vi "UI-电源尾反面标签漏线检测.vi"(8 "error in (no error)":errorcluster caption="错误输入（无错误）", 11 "名称或相对路径":string="Template Program") -> (0 "error in (no error) 2":errorcluster caption="错误输入（无错误）")   [LabVIEW 2017]
uses:
  Picture/SaveButtom.ctl
  Global System.vi
  <vilib>/Utility/xml.llb/Write to XML File(string).vi
panel:
  in  "获取图像":bool
  in  "ROI获取":bool
  in  "创建模板":bool
  in  "保存图像":bool
  out "添加的路径":path
  in  "刷新":bool
  in  "测试按钮":bool
  in  "保存按钮":bool
  in  "Main":enum32{"主参数", "颜色模板匹配参数 ", "测试效果"}(tab)
  in  "UI电源尾反面漏线基础参数":T1={"IsNorImage"=TRUE, "Exposure Values"=100289, "ImagePath"=path "C:/Users/hedongpo/Desktop/514-hdp/Alignment Assemble System/Test Picture/B/3.bmp"} caption="参数界面" {"Exposure Values" scale=0.0..200000.0}
  in  "UI电源尾反面漏线参数":T3={"Rectangle"={"Left"=0, "Top"=0, "Right"=0, "Bottom"=0, "Rotation"=0.0}, "模板路径"=path "C:/Users/delluser001/Desktop/PowerLine Inspect System/Source Code/Template Program/potteryTemplete/Color.png", "Match Mode "=0, "Minimum Match Score "=800.0, "Number of Matches Requested"=1, "Rotation Angle Ranges (degrees)"=[{"Min"=-180.0, "Max"=180.0}], "Color Sensitivity "=0, "Match Offset"={"X"=0.0, "Y"=0.0}, "Color Score Weight "=500.0, "Search Strategy "=0, "Subpixel Accuracy "=FALSE, "Range (Threshold 1)"={"Lower value"=148.0, "Upper value"=255.0}} {"Rectangle"."Rotation" format="%.2f"; "Rectangle"."Left" scale=0.0..1024.0; "Rectangle"."Right" scale=0.0..1024.0; "Search Strategy" items=["Conservative", "Balance", "Aggressive", "Very Aggressive"]; "Color Sensitivity" items=["Low Sensitivity", "Medium Sensitivity", "High Sensitivity"]; "Match Mode" items=["Shift Invariant", "Rotation Invariant"]}
  out "原始图像":T4(plugin-control)
  out "x = 0?":bool
  out "路径输出":path
  in  "Vision Paramter Save Buttom":T5
  out "system time":string
  in  "取消按钮":bool
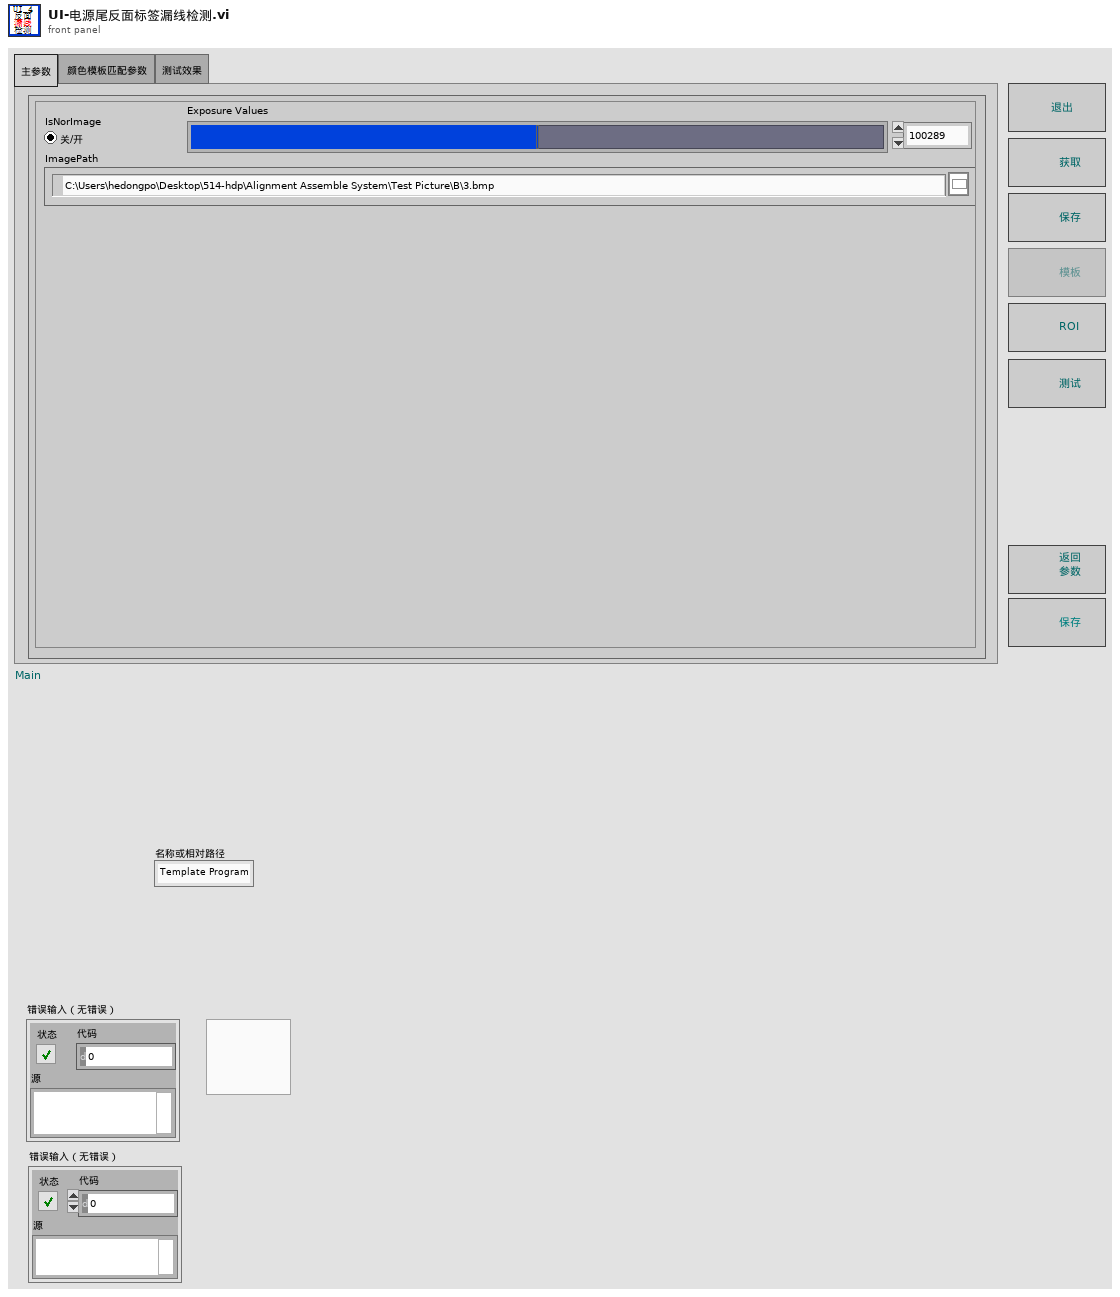
[diagram p1: front panel]
types:
  T1 = cluster{"IsNorImage":bool, "Exposure Values":u32, "ImagePath":path}
  T2 = typedef "IMAQ Rectangle" = cluster{"Left":i32, "Top":i32, "Right":i32, "Bottom":i32, "Rotation":dbl}
  T3 = cluster{"Rectangle":T2, "模板路径":path, "Match Mode ":u32, "Minimum Match Score ":sgl, "Number of Matches Requested":i32, "Rotation Angle Ranges (degrees)":cluster{"Min":sgl, "Max":sgl}[], "Color Sensitivity ":u32, "Match Offset":cluster{"X":sgl, "Y":sgl}, "Color Score Weight ":sgl, "Search Strategy ":u32, "Subpixel Accuracy ":bool, "Range (Threshold 1)":cluster{"Lower value":sgl, "Upper value":sgl}}
  T4 = typedef "IMAQ Image.ctl" = refnum<image>
  T5 = typedef "SaveButtom.ctl" = bool
  T6 = cluster{"index":i32, "this vi":refnum<vi>, "error out":errorcluster}
  T7 = cluster{"master data":string, "priority":u16, "secondary data":string[]}
  T8 = cluster{"case name":string[], "queue array":refnum<queue>[]}
  T9 = cluster{"Global Rectangle":i32[], "Contours":cluster{"Contour Type":u32, "ROI Type":u32, "Points":i32[]}[]}
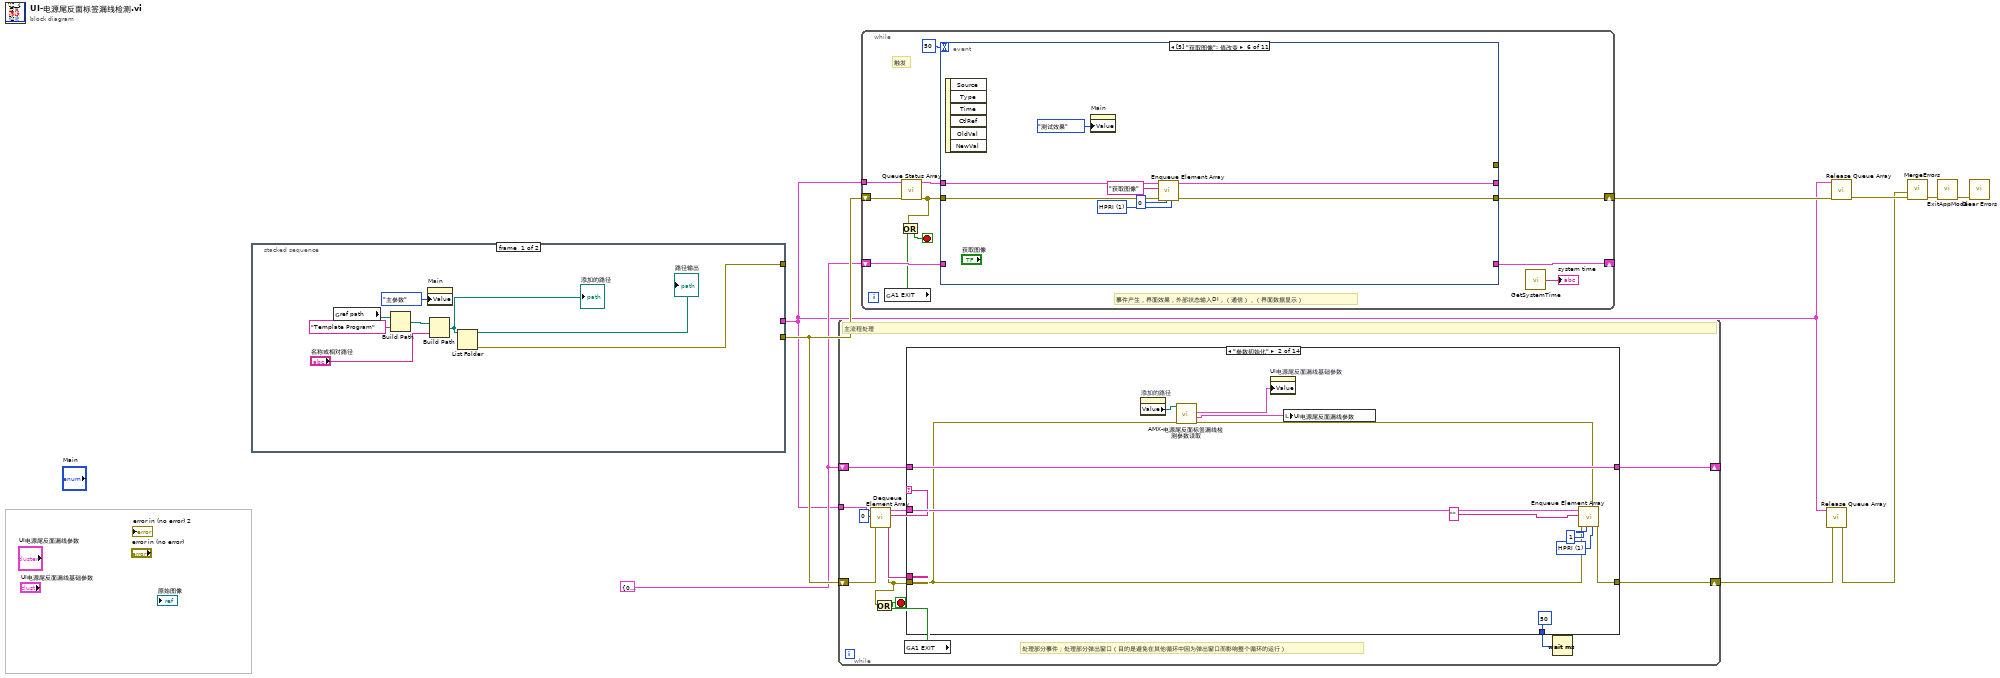
[diagram p0: block diagram]
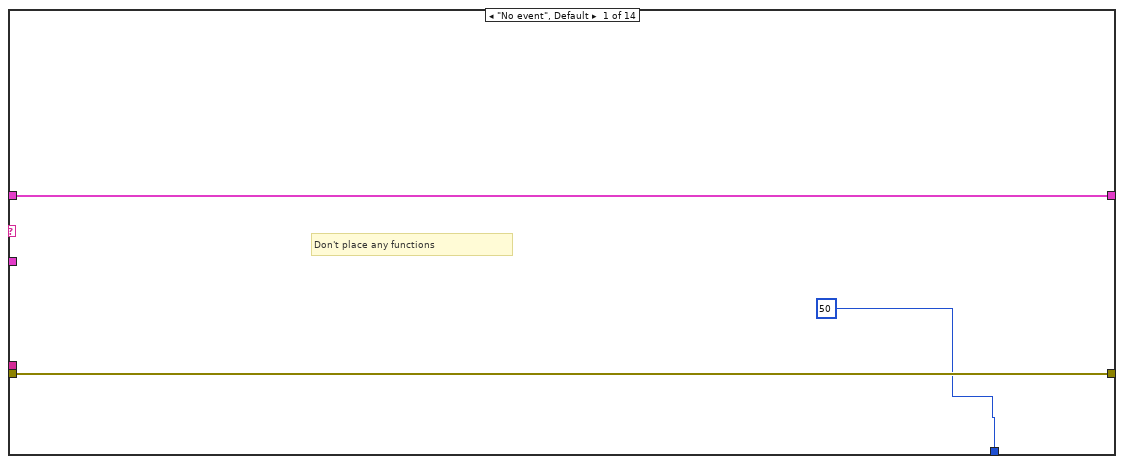
[diagram p2: hidden frame]
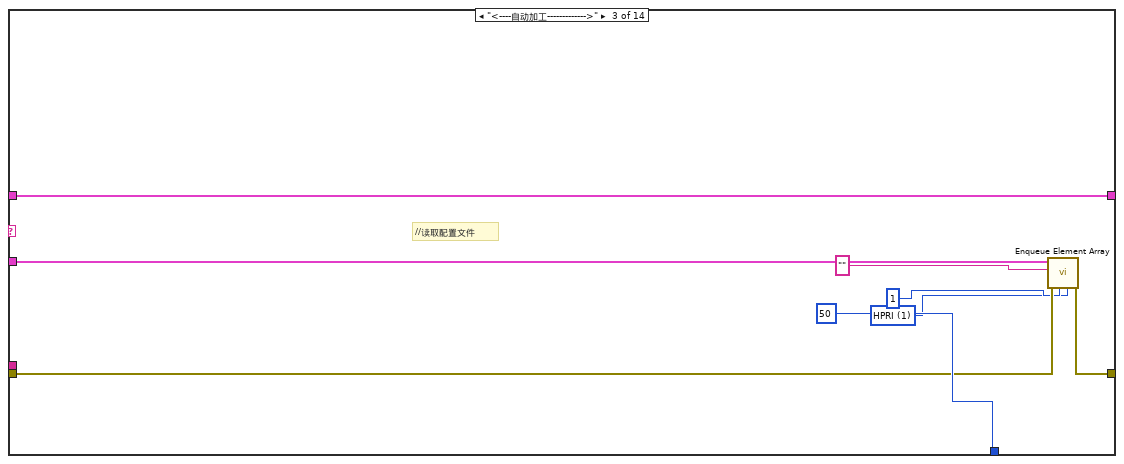
[diagram p3: hidden frame]
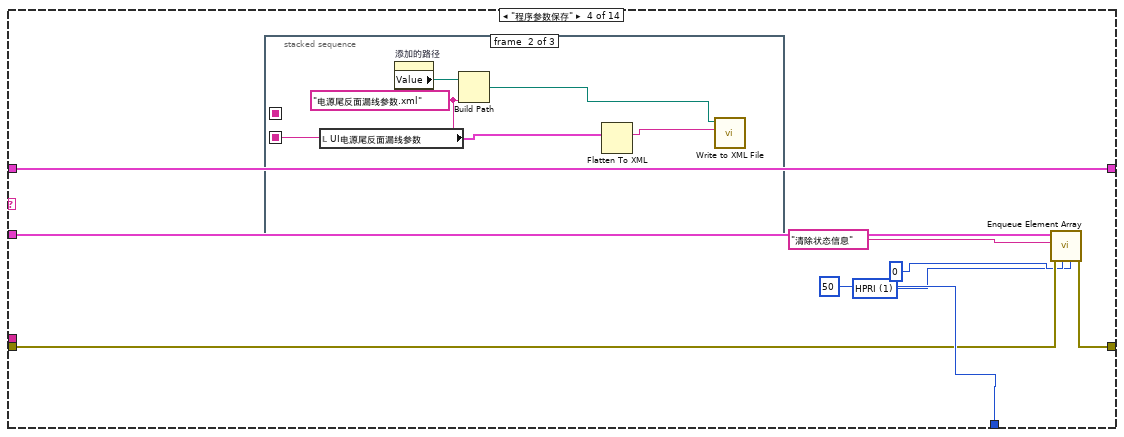
[diagram p4: hidden frame]
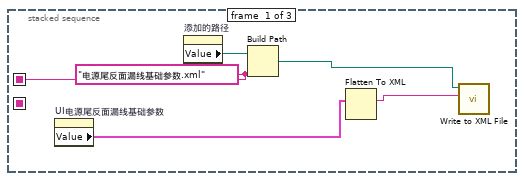
[diagram p5: hidden frame]
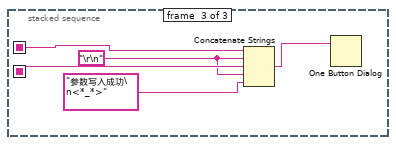
[diagram p6: hidden frame]
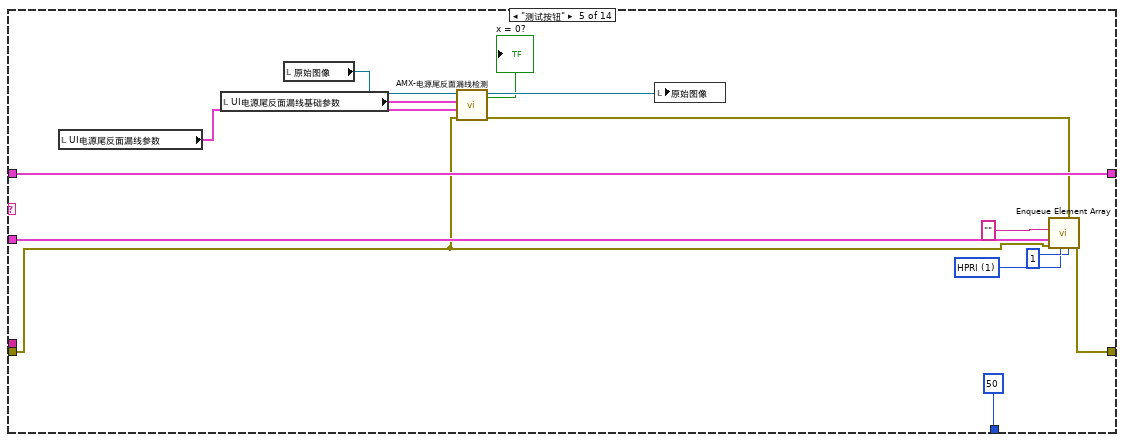
[diagram p7: hidden frame]
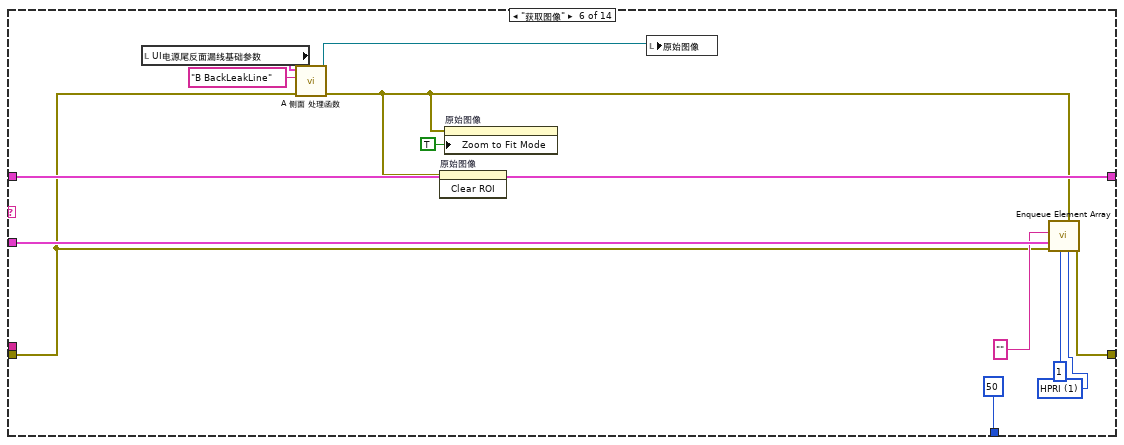
[diagram p8: hidden frame]
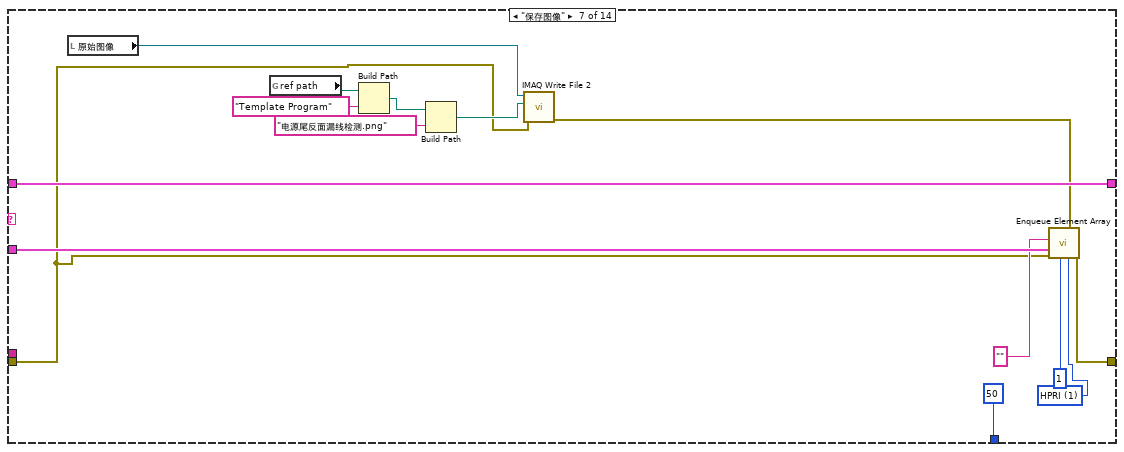
[diagram p9: hidden frame]
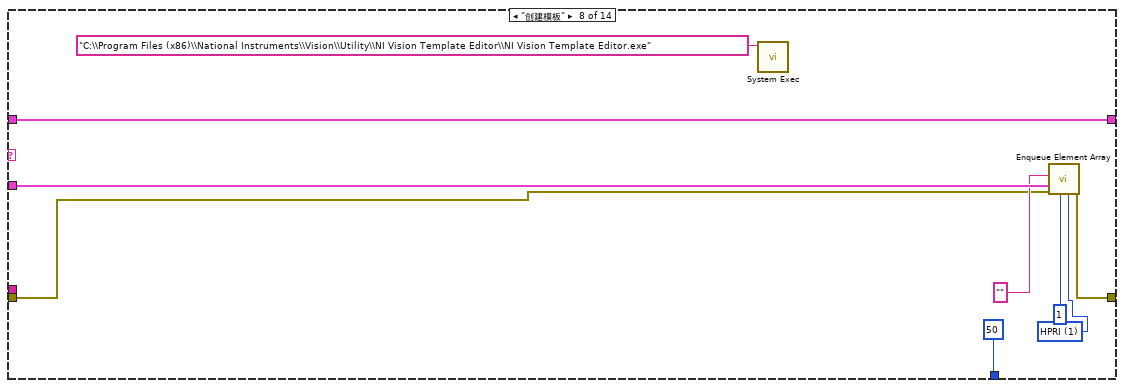
[diagram p10: hidden frame]
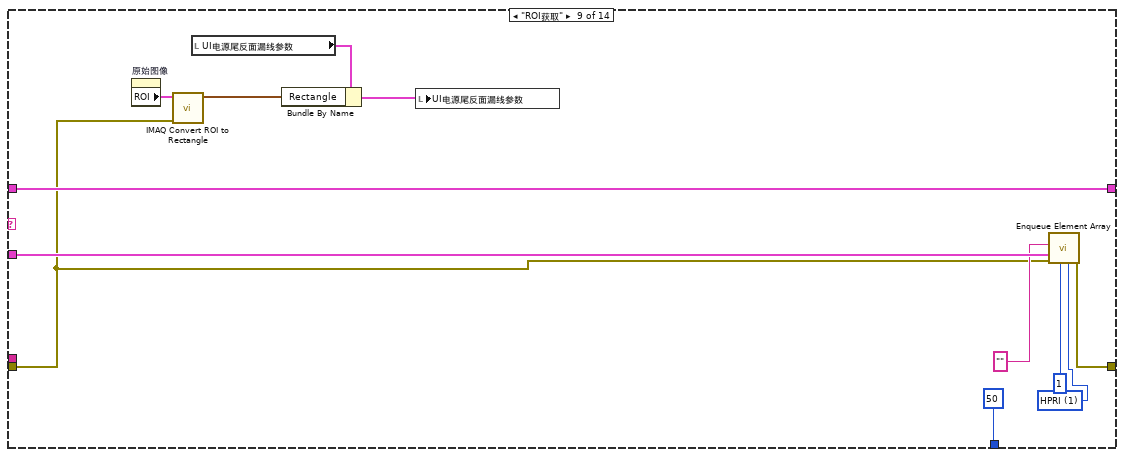
[diagram p11: hidden frame]
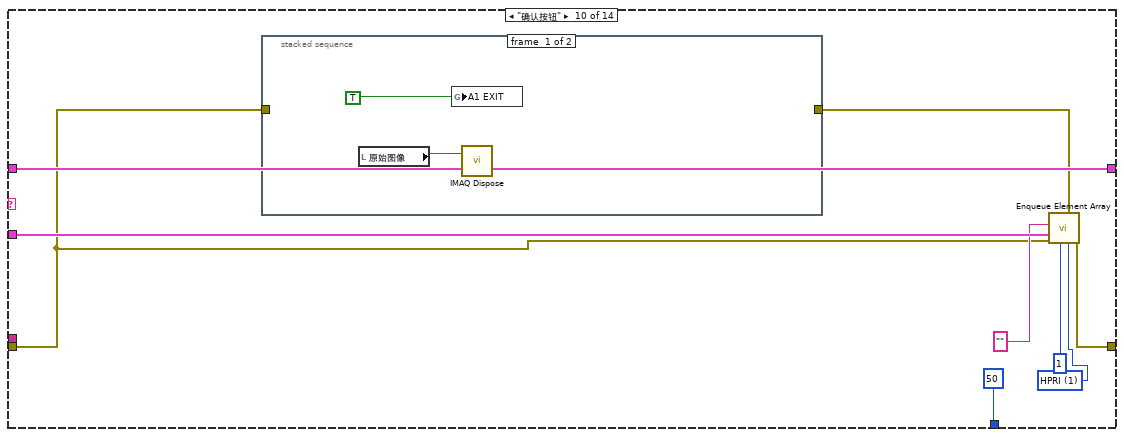
[diagram p12: hidden frame]
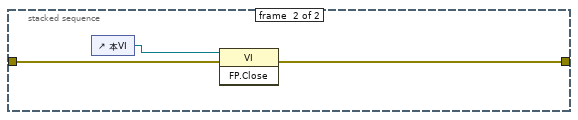
[diagram p13: hidden frame]
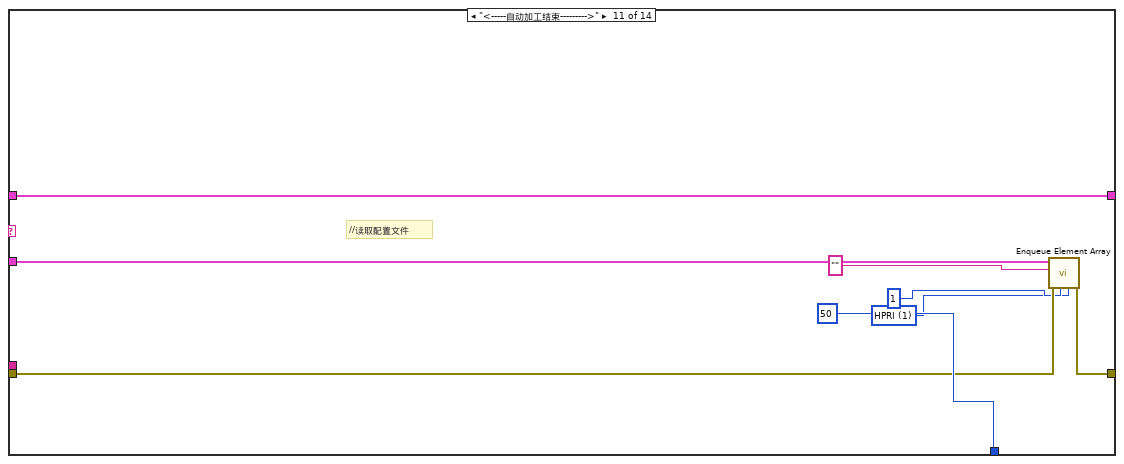
[diagram p14: hidden frame]
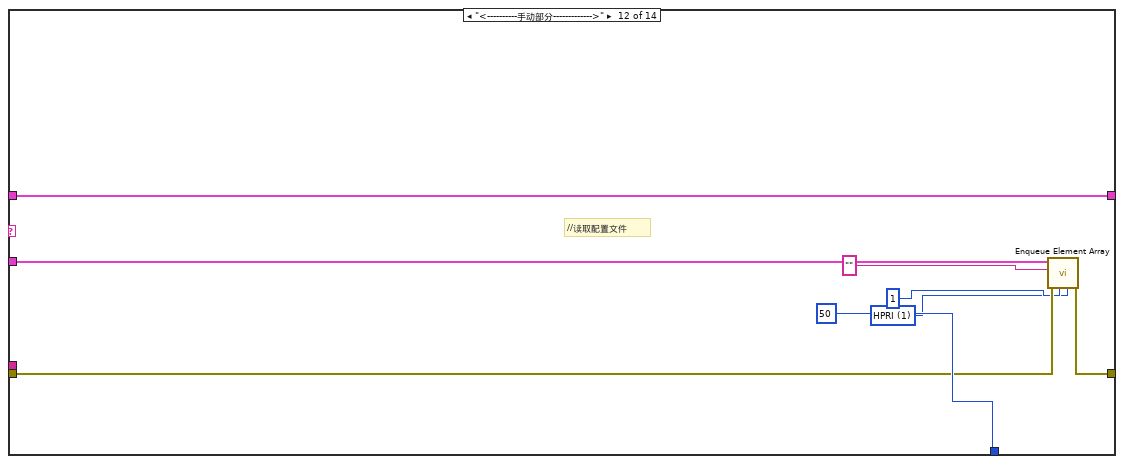
[diagram p15: hidden frame]
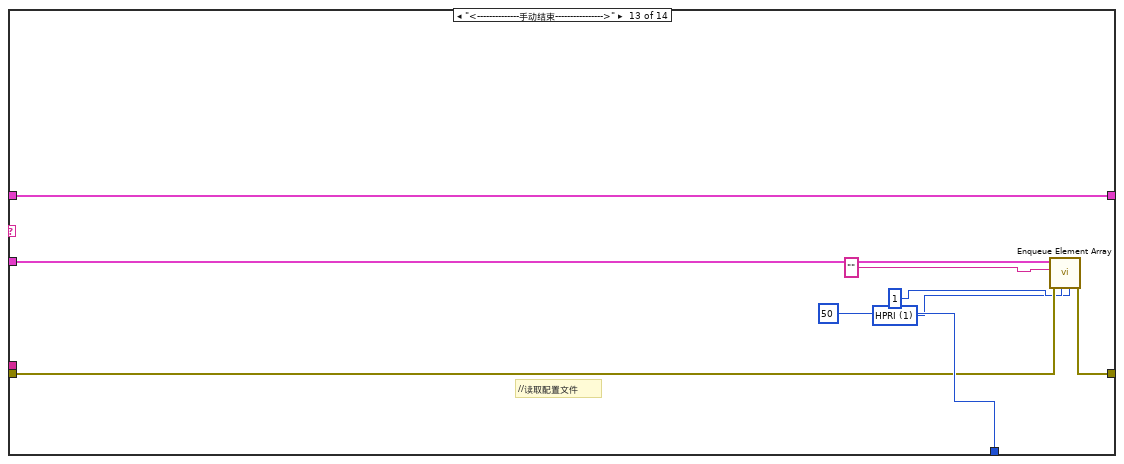
[diagram p16: hidden frame]
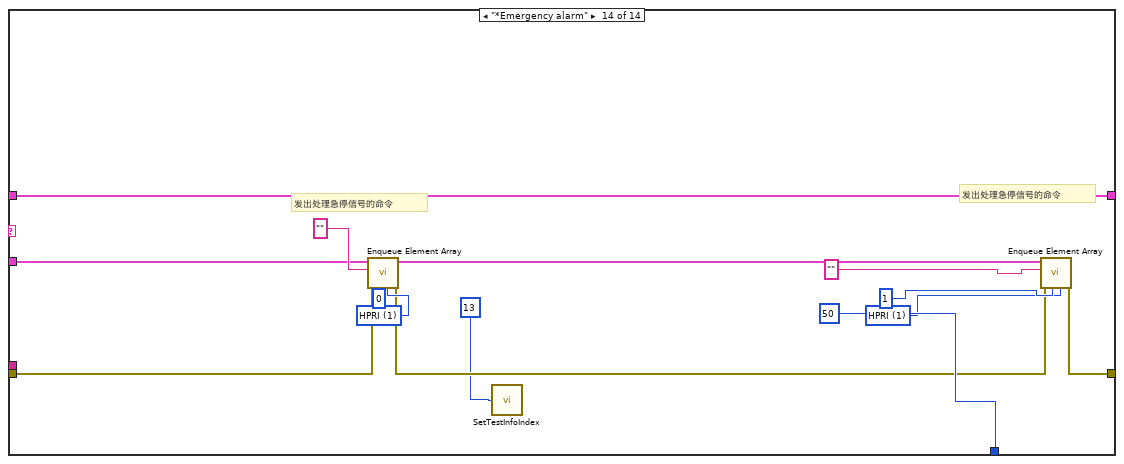
[diagram p17: hidden frame]
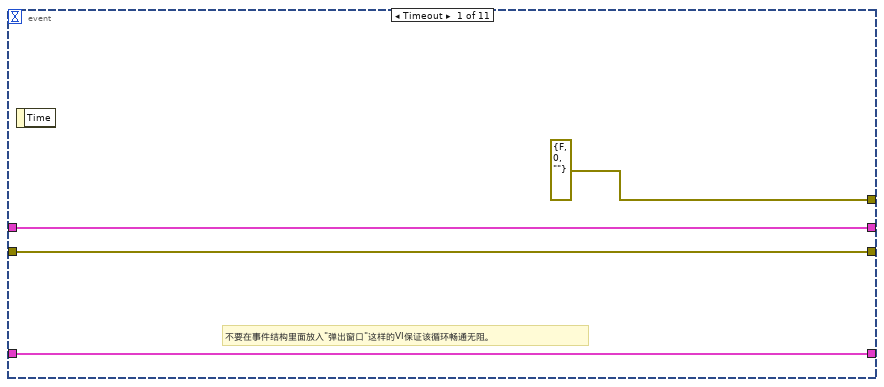
[diagram p18: hidden frame]
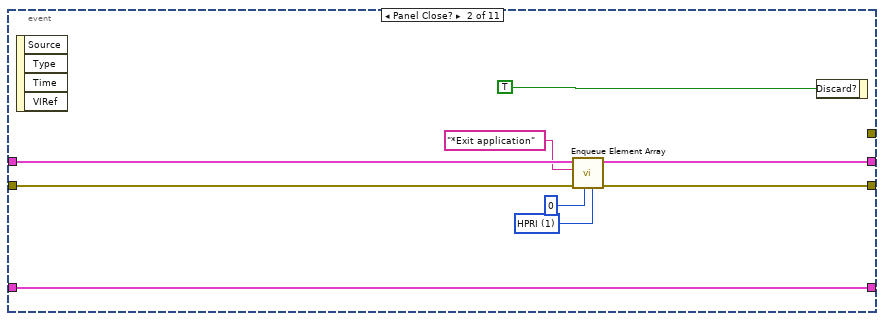
[diagram p19: hidden frame]
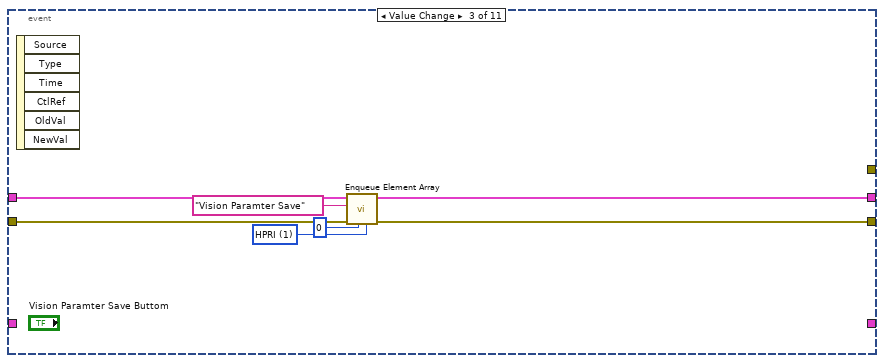
[diagram p20: hidden frame]
diagram:
  w4 = T6 {"index"=0, "this vi"=refnum, "error out"={"status"=FALSE, "code"=0, "source"=""}} ("parameter buffer")
  n1 = stacked-sequence {
    tunnel: [w16 _] -> _
    tunnel: [_ w19] -> w5
    tunnel: [_ w18] -> w1
    frame #0 {
      n2 = global read "Global System.vi" "ref path"() -> (w14:path)
      n3 = Build Path(base path=w14, name or relative path="Template Program" ("名称或相对路径")) -> (appended path=w12:path)
      n4 = property on="Main" class="TabCtl (严格)"("Value"=enum32{"主参数", "颜色模板匹配参数 ", "测试效果"}."主参数" ("Main")) -> ()  [unwired: 2 in, 2 out]
      n5 = Build Path(base path=w12, name or relative path="名称或相对路径") -> (appended path=w10:path)
      "添加的路径" <- w10
      n6 = List Folder(path=w10) -> (path out=→"路径输出":path, error out=w16:errorcluster)  [unwired: 3 in, 2 out]
    }
    frame #1 {
      w27 = string[] ["comm queue1", "data queue 11", "data queue 12", "data queue 13", "data queue 14"]  # queue name
      w28 = 4  # queue num
      w29 = T7 {"master data"="", "priority"=0, "secondary data"=[]}  # element data type
      n7 = call "Obtain Queue Array.vi"("queue name"=w27, "element data type"=w29, "queue num"=w28) -> ("error out"=w23:errorcluster, "queue out"=w24:T8)  [unwired: 2 in, 1 out]
      n8 = call "Enqueue Element Array.vi"("queue index"=0, "error in"=w23, "master data"="参数初始化", "queue in"=w24) -> ("error out"=w22:errorcluster, "queue out"=w21:T8)  [unwired: 6 in]
      n9 = disable-structure shown="启用" {
        disable-tunnel: w22 -> [w35 w36]
        disable-tunnel: w21 -> [w34 w37]
        disable-tunnel: "Loading Variable" ("master data") -> [w33 _]
        disable-tunnel: [w31 w36] -> w19
        disable-tunnel: [w30 w37] -> w18
        frame Disabled {
          n10 = call "Enqueue Element Array.vi"("queue index"=12, "error in"=w35, "master data"=w33, "queue in"=w34) -> ("error out"=w31:errorcluster, "queue out"=w30:T8)  [unwired: 6 in]
        }
        frame Enabled {
        }
      }
    }
  }
  n11 = while {
    shift-right: [w50] -> w3
    shift-left: w5 -> [w41]
    shift-right: [w47] -> _
    shift-left: w4 -> [w48]
    tunnel: w1 -> [w43]
    stop <- w38 stop-if-true
    # "处理部分事件；处理部分弹出窗口（目的是避免在其他循环中因为弹出窗口而影响整个循环的运行）"
    # "主流程处理"
    n12 = call "Dequeue Element Array.vi"("queue in"=w43, "queue index"=0, "error in"=w41) -> ("queue out"=w46:T8, "master data"=w45:string, "secondary data"=w44:string[], "error out"=w40:errorcluster)  [unwired: 2 in, 1 out]
    n13 = global read "Global System.vi" "A1 EXIT"() -> (w39:bool)
    n14 = Or(x=w40, y=w39) -> (x .or. y?=w38:bool)
    n15 = case shown="\"参数初始化\"" w45 {
      tunnel: w46 -> [_ w64 w72 w74 w109 w122 w137 w146 w158 w167 w180 w188 w196 w202]
      tunnel: w40 -> [w52 w57 w68 w78 w102 w113 w124 w140 w151 w161 w176 w184 w192 w199]
      tunnel: [w52 w63 w71 w80 w108 w121 w136 w145 w157 w166 w179 w187 w195 w210] -> w50
      tunnel: [50 50 50 50 50 50 50 50 50 50 50 50 50 50] -> w49
      tunnel: w48 -> [w53 w59 w69 w75 w104 w117 w132 w141 w153 w162 w177 w185 w193 w208]
      tunnel: [w53 w59 w69 w75 w104 w117 w132 w141 w153 w162 w177 w185 w193 w208] -> w47
      tunnel: w44 -> [_ _ _ _ _ _ _ _ _ _ _ _ _ _]
      frame "No event", Default {
        # "Don't place any functions"
      }
      frame "参数初始化" {
        w60 = u16 1 items=["HPRI"=1, "LPRI"=0] ("priority")
        n16 = property on="添加的路径" class="Path"() -> ("Value"=w58:path)  [unwired: 2 in, 2 out]
        n17 = call "AMX-电源尾反面标签漏线检测参数读取.vi"("error in (no error)"=w57, "基路径"=w58) -> ("error out"=w55:errorcluster, "UI电源尾反面漏线参数"=w54:T3, "UI电源尾反面漏线基础参数"=w56:T1)  [unwired: 6 in]
        n18 = property on="UI电源尾反面漏线基础参数" class="Clust (严格)"("Value"=w56) -> ()  [unwired: 2 in, 2 out]
        n19 = local write "UI电源尾反面漏线参数"(w54) -> ()
        n20 = call "Enqueue Element Array.vi"("priority"=w60, "device error in"=w55, "queue index"=1, "error in"=w57, "master data"="" ("Element 1"), "queue in"=w64) -> ("error out"=w63:errorcluster)  [unwired: 4 in, 1 out]
      }
      frame "<----自动加工------------->" {
        w66 = u16 1 items=["HPRI"=1, "LPRI"=0] ("priority")
        # "//读取配置文件"
        n21 = call "Enqueue Element Array.vi"("priority"=w66, "queue index"=1, "error in"=w68, "master data"="" ("Element 1"), "queue in"=w72) -> ("error out"=w71:errorcluster)  [unwired: 5 in, 1 out]
      }
      frame "程序参数保存" {
        w76 = u16 1 items=["HPRI"=1, "LPRI"=0] ("priority")
        n22 = stacked-sequence {
          seq-local: [w82 _ _] -> [_ _ w95]
          seq-local: [_ w88 _] -> [_ _ w93]
          frame #0 {
            w82 = "电源尾反面漏线基础参数.xml" ("名称或相对路径")
            n23 = property on="UI电源尾反面漏线基础参数" class="Clust (严格)"() -> ("Value"=w85:T1)  [unwired: 2 in, 2 out]
            n24 = property on="添加的路径" class="Path"() -> ("Value"=w86:path)  [unwired: 2 in, 2 out]
            n25 = Build Path(base path=w86, name or relative path=w82) -> (appended path=w83:path)
            n26 = Flatten To XML(anything=w85) -> (xml string=w84:string)
            n27 = call-poly <vilib>:"Write to XML File.vi"("XML Input"=w84, "XML File Path"=w83) -> ()  [unwired: 7 in, 3 out]
          }
          frame #1 {
            w88 = "电源尾反面漏线参数.xml" ("名称或相对路径")
            n28 = local read "UI电源尾反面漏线参数"() -> (w87:T3)
            n29 = property on="添加的路径" class="Path"() -> ("Value"=w91:path)  [unwired: 2 in, 2 out]
            n30 = Build Path(base path=w91, name or relative path=w88) -> (appended path=w89:path)
            n31 = Flatten To XML(anything=w87) -> (xml string=w90:string)
            n32 = call-poly <vilib>:"Write to XML File.vi"("XML Input"=w90, "XML File Path"=w89) -> ()  [unwired: 7 in, 3 out]
          }
          frame #2 {
            w92 = "\r\n"
            n33 = Concatenate Strings(w95, w92, w93, w92, "参数写入成功\n<*_*>" ("消息")) -> (w94:string)
            n34 = One Button Dialog(message=w94) -> ()  [unwired: 1 in, 1 out]
          }
        }
        n35 = call "Enqueue Element Array.vi"("priority"=w76, "queue index"=0, "error in"=w78, "master data"="清除状态信息" ("Element 1"), "queue in"=w74) -> ("error out"=w80:errorcluster)  [unwired: 5 in, 1 out]
      }
      frame "测试按钮" {
        w105 = u16 1 items=["HPRI"=1, "LPRI"=0] ("priority")
        n36 = local read "UI电源尾反面漏线参数"() -> (w98:T3)
        n37 = local read "UI电源尾反面漏线基础参数"() -> (w103:T1)
        n38 = local read "原始图像"() -> (w100:T4)
        n39 = call "AMX-电源尾反面漏线检测.vi"("error in (no error)"=w102, "UI电源线正面漏线参数"=w98, "电源线正面标签1基础参数"=w103, "Image in"=w100) -> ("error out"=w99:errorcluster, "Image out"=w101:T4, "x = 0?"=→"x = 0?":bool)  [unwired: 5 in]
        n40 = local write "原始图像"(w101) -> ()
        n41 = call "Enqueue Element Array.vi"("priority"=w105, "device error in"=w99, "queue index"=1, "error in"=w102, "master data"="" ("Element 1"), "queue in"=w109) -> ("error out"=w108:errorcluster)  [unwired: 4 in, 1 out]
      }
      frame "获取图像" {
        w118 = u16 1 items=["HPRI"=1, "LPRI"=0] ("priority")
        n42 = local read "UI电源尾反面漏线基础参数"() -> (w115:T1)
        n43 = call "A 侧面 处理函数.vi"("error in (no error)"=w113, "Image Name"="B BackLeakLine", "ParamsUI"=w115) -> ("error out"=w111:errorcluster, "Image out"=w114:T4)  [unwired: 5 in, 2 out]
        n44 = invoke on="原始图像" class="ImageControl" method="Clear ROI"(error in=w111) -> ()  [unwired: 2 in, 3 out]
        n45 = property on="原始图像" class="ImageControl"(error in=w111, "Zoom to Fit Mode"=TRUE) -> ()  [unwired: 1 in, 2 out]
        n46 = local write "原始图像"(w114) -> ()
        n47 = call "Enqueue Element Array.vi"("priority"=w118, "device error in"=w111, "queue index"=1, "error in"=w113, "master data"="" ("Element 1"), "queue in"=w122) -> ("error out"=w121:errorcluster)  [unwired: 4 in, 1 out]
      }
      frame "保存图像" {
        w133 = u16 1 items=["HPRI"=1, "LPRI"=0] ("priority")
        n48 = local read "原始图像"() -> (w125:T4)
        n49 = global read "Global System.vi" "ref path"() -> (w131:path)
        n50 = Build Path(base path=w131, name or relative path="Template Program" ("名称或相对路径")) -> (appended path=w129:path)
        n51 = Build Path(base path=w129, name or relative path="电源尾反面漏线检测.png" ("名称或相对路径")) -> (appended path=w127:path)
        n52 = call-poly "IMAQ Write File 2"("error in (no error)"=w124, "File Path"=w127, "Image"=w125) -> ("error out"=w126:errorcluster)  [unwired: 7 in, 1 out]
        n53 = call "Enqueue Element Array.vi"("priority"=w133, "device error in"=w126, "queue index"=1, "error in"=w124, "master data"="" ("Element 1"), "queue in"=w137) -> ("error out"=w136:errorcluster)  [unwired: 4 in, 1 out]
      }
      frame "创建模板" {
        w142 = u16 1 items=["HPRI"=1, "LPRI"=0] ("priority")
        n54 = call <vilib>:"System Exec.vi"("command line"="C:\\Program Files (x86)\\National Instruments\\Vision\\Utility\\NI Vision Template Editor\\NI Vision Template Editor.exe") -> ()  [unwired: 7 in, 4 out]
        n55 = call "Enqueue Element Array.vi"("priority"=w142, "queue index"=1, "error in"=w140, "master data"="" ("Element 1"), "queue in"=w146) -> ("error out"=w145:errorcluster)  [unwired: 5 in, 1 out]
      }
      frame "ROI获取" {
        w154 = u16 1 items=["HPRI"=1, "LPRI"=0] ("priority")
        n56 = property on="原始图像" class="ImageControl"() -> ("ROI"=w152:T9)  [unwired: 2 in, 2 out]
        n57 = call "IMAQ Convert ROI to Rectangle"("error in (no error)"=w151, "ROI Descriptor"=w152) -> ("Rectangle"=w149:T2)  [unwired: 7 in, 1 out]
        n58 = local read "UI电源尾反面漏线参数"() -> (w150:T3)
        n59 = Bundle By Name(cluster=w150, "Rectangle"=w149) -> (w148:T3)
        n60 = local write "UI电源尾反面漏线参数"(w148) -> ()
        n61 = call "Enqueue Element Array.vi"("priority"=w154, "queue index"=1, "error in"=w151, "master data"="" ("Element 1"), "queue in"=w158) -> ("error out"=w157:errorcluster)  [unwired: 5 in, 1 out]
      }
      frame "确认按钮" {
        w163 = u16 1 items=["HPRI"=1, "LPRI"=0] ("priority")
        n62 = stacked-sequence {
          tunnel: w161 -> [_ w172]
          tunnel: [_ w171] -> w160
          frame #0 {
            n63 = local read "原始图像"() -> (w169:T4)
            n64 = global write "Global System.vi" "A1 EXIT"(TRUE ("EXIT")) -> ()
            n65 = call "IMAQ Dispose"("Image"=w169) -> ()  [unwired: 5 in, 1 out]
          }
          frame #1 {
            n66 = control-ref of="本VI"() -> (w173:refnum<vi>)
            n67 = invoke class="VI" method="FP.Close"(reference=w173, error in=w172) -> (error out=w171:errorcluster)  [unwired: 1 in, 2 out]
          }
        }
        n68 = call "Enqueue Element Array.vi"("priority"=w163, "device error in"=w160, "queue index"=1, "error in"=w161, "master data"="" ("Element 1"), "queue in"=w167) -> ("error out"=w166:errorcluster)  [unwired: 4 in, 1 out]
      }
      frame "<-----自动加工结束--------->" {
        w174 = u16 1 items=["HPRI"=1, "LPRI"=0] ("priority")
        # "//读取配置文件"
        n69 = call "Enqueue Element Array.vi"("priority"=w174, "queue index"=1, "error in"=w176, "master data"="" ("Element 1"), "queue in"=w180) -> ("error out"=w179:errorcluster)  [unwired: 5 in, 1 out]
      }
      frame "<----------手动部分------------->" {
        w182 = u16 1 items=["HPRI"=1, "LPRI"=0] ("priority")
        # "//读取配置文件"
        n70 = call "Enqueue Element Array.vi"("priority"=w182, "queue index"=1, "error in"=w184, "master data"="" ("Element 1"), "queue in"=w188) -> ("error out"=w187:errorcluster)  [unwired: 5 in, 1 out]
      }
      frame "<--------------手动结束---------------->" {
        w190 = u16 1 items=["HPRI"=1, "LPRI"=0] ("priority")
        # "//读取配置文件"
        n71 = call "Enqueue Element Array.vi"("priority"=w190, "queue index"=1, "error in"=w192, "master data"="" ("Element 1"), "queue in"=w196) -> ("error out"=w195:errorcluster)  [unwired: 5 in, 1 out]
      }
      frame "*Emergency alarm" {
        w205 = u16 1 items=["HPRI"=1, "LPRI"=0] ("priority")
        w206 = u16 1 items=["HPRI"=1, "LPRI"=0] ("priority")
        # "发出处理急停信号的命令"
        # "发出处理急停信号的命令"
        n72 = call "Enqueue Element Array.vi"("priority"=w205, "queue index"=0, "error in"=w199, "master data"="" ("Element 1"), "queue in"=w202) -> ("error out"=w200:errorcluster, "queue out"=w201:T8)  [unwired: 5 in]
        n73 = call "SetTestInfoIndex.vi"("test info index"=13) -> ()
        n74 = call "Enqueue Element Array.vi"("priority"=w206, "queue index"=1, "error in"=w200, "master data"="" ("Element 1"), "queue in"=w201) -> ("error out"=w210:errorcluster)  [unwired: 5 in, 1 out]
      }
    }
    n75 = Wait (ms)(milliseconds to wait=w49) -> ()  [unwired: 1 out]
  }
  n76 = while {
    shift-right: [w215] -> w6
    shift-left: w5 -> [w219]
    shift-right: [w217] -> _
    shift-left: w4 -> [w218]
    tunnel: w1 -> [w221]
    stop <- w212 stop-if-true
    # "触发"
    # "事件产生，界面效果，外部状态输入DI，（通信），（界面数据显示）"
    n77 = global read "Global System.vi" "A1 EXIT"() -> (w213:bool)
    n78 = call "Queue Status Array.vi"("error in (no error)"=w219, "queue in"=w221) -> ("error out"=w214:errorcluster, "queue out"=w216:T8)  [unwired: 4 in]
    n79 = Or(x=w214, y=w213) -> (x .or. y?=w212:bool)
    n80 = event shown="[5] \"获取图像\": 值改变" {
      selector: _ -> [_ _ _ _ _ _ _ _ _ _ _]
      dyn-events: _ -> [_ _ _ _ _ _ _ _ _ _ _]
      timeout: 50 -> [_ _ _ _ _ _ _ _ _ _ _]
      tunnel: w218 -> [w226 w234 _ _ _ _ _ _ _ _ _]
      tunnel: [w226 w234 _ _ _ _ _ _ _ _ _] -> w217
      tunnel: [errorcluster {"status"=FALSE, "code"=0, "source"=""} ("error out") _ _ _ _ _ _ _ _ _ _] -> _
      tunnel: w216 -> [w224 w233 w239 w246 w253 w261 w268 w275 w283 w291 w299]
      tunnel: w214 -> [w223 w232 w238 w245 w252 w260 w267 w274 w282 w290 w298]
      tunnel: [w223 w231 w236 w243 w250 w258 w265 w272 w280 w288 w296] -> w215
      tunnel: [w224 w230 w237 w244 w251 w259 w266 w273 w281 w289 w297] -> _
      event Timeout {
        # "不要在事件结构里面放入\"弹出窗口\"这样的VI保证该循环畅通无阻。"
        n81 = event-data() -> ()  [unwired: 1 in, 1 out]
      }
      event Panel Close? {
        w228 = u16 1 items=["HPRI"=1, "LPRI"=0] ("priority")
        n82 = event-data() -> ()  [unwired: 1 in, 4 out]
        n83 = call "Enqueue Element Array.vi"("priority"=w228, "queue index"=0, "error in"=w232, "master data"="*Exit application", "queue in"=w233) -> ("error out"=w231:errorcluster, "queue out"=w230:T8)  [unwired: 5 in]
        n84 = event-data("Discard?"=TRUE) -> ()  [unwired: 1 in, 1 out]
      }
      event Value Change {
        w241 = u16 1 items=["HPRI"=1, "LPRI"=0] ("priority")
        n85 = event-data() -> ()  [unwired: 1 in, 6 out]
        n86 = call "Enqueue Element Array.vi"("priority"=w241, "queue index"=0, "error in"=w238, "master data"="Vision Paramter Save", "queue in"=w239) -> ("error out"=w236:errorcluster, "queue out"=w237:T8)  [unwired: 5 in]
      }
      event "取消按钮": Value Change {
        w248 = u16 1 items=["HPRI"=1, "LPRI"=0] ("priority")
        n87 = event-data() -> ()  [unwired: 1 in, 6 out]
        n88 = call "Enqueue Element Array.vi"("priority"=w248, "queue index"=0, "error in"=w245, "master data"="确认按钮", "queue in"=w246) -> ("error out"=w243:errorcluster, "queue out"=w244:T8)  [unwired: 5 in]
      }
      event "保存按钮": Value Change {
        w255 = u16 1 items=["HPRI"=1, "LPRI"=0] ("priority")
        n89 = event-data() -> ()  [unwired: 1 in, 6 out]
        n90 = call "Enqueue Element Array.vi"("priority"=w255, "queue index"=0, "error in"=w252, "master data"="程序参数保存", "queue in"=w253) -> ("error out"=w250:errorcluster, "queue out"=w251:T8)  [unwired: 5 in]
      }
      event "获取图像": Value Change {
        w263 = u16 1 items=["HPRI"=1, "LPRI"=0] ("priority")
        n91 = event-data() -> ()  [unwired: 1 in, 6 out]
        n92 = property on="Main" class="TabCtl (严格)"("Value"=enum32{"主参数", "颜色模板匹配参数 ", "测试效果"}."测试效果" ("Main")) -> ()  [unwired: 2 in, 2 out]
        n93 = call "Enqueue Element Array.vi"("priority"=w263, "queue index"=0, "error in"=w260, "master data"="获取图像", "queue in"=w261) -> ("error out"=w258:errorcluster, "queue out"=w259:T8)  [unwired: 5 in]
      }
      event "保存图像": Value Change {
        w270 = u16 1 items=["HPRI"=1, "LPRI"=0] ("priority")
        n94 = event-data() -> ()  [unwired: 1 in, 6 out]
        n95 = call "Enqueue Element Array.vi"("priority"=w270, "queue index"=0, "error in"=w267, "master data"="保存图像", "queue in"=w268) -> ("error out"=w265:errorcluster, "queue out"=w266:T8)  [unwired: 5 in]
      }
      event "创建模板": Value Change {
        w277 = u16 1 items=["HPRI"=1, "LPRI"=0] ("priority")
        n96 = event-data() -> ()  [unwired: 1 in, 6 out]
        n97 = call "Enqueue Element Array.vi"("priority"=w277, "queue index"=0, "error in"=w274, "master data"="创建模板", "queue in"=w275) -> ("error out"=w272:errorcluster, "queue out"=w273:T8)  [unwired: 5 in]
      }
      event "ROI获取": Value Change {
        w285 = u16 1 items=["HPRI"=1, "LPRI"=0] ("priority")
        n98 = event-data() -> ()  [unwired: 1 in, 6 out]
        n99 = property on="Main" class="TabCtl (严格)"("Value"=enum32{"主参数", "颜色模板匹配参数 ", "测试效果"}."颜色模板匹配参数 " ("Main")) -> ()  [unwired: 2 in, 2 out]
        n100 = call "Enqueue Element Array.vi"("priority"=w285, "queue index"=0, "error in"=w282, "master data"="ROI获取", "queue in"=w283) -> ("error out"=w280:errorcluster, "queue out"=w281:T8)  [unwired: 5 in]
      }
      event "测试按钮": Value Change {
        w293 = u16 1 items=["HPRI"=1, "LPRI"=0] ("priority")
        n101 = event-data() -> ()  [unwired: 1 in, 6 out]
        n102 = property on="Main" class="TabCtl (严格)"("Value"=enum32{"主参数", "颜色模板匹配参数 ", "测试效果"}."测试效果" ("Main")) -> ()  [unwired: 2 in, 2 out]
        n103 = call "Enqueue Element Array.vi"("priority"=w293, "queue index"=0, "error in"=w290, "master data"="测试按钮", "queue in"=w291) -> ("error out"=w288:errorcluster, "queue out"=w289:T8)  [unwired: 5 in]
      }
      event "刷新": Value Change {
        n104 = event-data() -> ()  [unwired: 1 in, 6 out]
        n105 = disable-structure shown="禁用" {
          disable-tunnel: w299 -> [w303 _]
          disable-tunnel: w298 -> [w302 _]
          disable-tunnel: [w301 _] -> w297
          disable-tunnel: [w300 _] -> w296
          frame Disabled {
            w305 = u16 1 items=["HPRI"=1, "LPRI"=0] ("priority")
            # "刷新"
            n106 = call "Enqueue Element Array.vi"("priority"=w305, "queue index"=0, "error in"=w302, "master data"="刷新", "queue in"=w303) -> ("error out"=w300:errorcluster, "queue out"=w301:T8)  [unwired: 5 in]
          }
          frame Enabled {
          }
        }
        n107 = property on="Main" class="TabCtl (严格)"("Value"=enum32{"主参数", "颜色模板匹配参数 ", "测试效果"}."颜色模板匹配参数 " ("Main")) -> ()  [unwired: 2 in, 2 out]
      }
    }
    n108 = call "GetSystemTime.vi"() -> ("date/time string"=→"system time":string)  [unwired: 7 in]
  }
  n109 = call "Release Queue Array.vi"("error in"=w3, "queue in"=w1) -> ("error out"=w2:errorcluster)  [unwired: 2 in, 3 out]
  n110 = call "Release Queue Array.vi"("error in"=w6, "queue in"=w1) -> ("error out"=w9:errorcluster)  [unwired: 2 in, 3 out]
  n111 = call "MergeErrors.vi"("error in 3 (no error)"=w2, "error in 4 (no error)"=w9) -> ("error out"=w8:errorcluster)  [unwired: 6 in]
  n112 = call "ExitAppMode.vi"("error in (no error)"=w8) -> ("error out"=w7:errorcluster)  [unwired: 10 in]
  n113 = call <vilib>:"Clear Errors.vi"("error in (no error)"=w7) -> ()  [unwired: 5 in, 2 out]
